vi "donut_fitting_particle(subVI).vi"(5 "Edge Options":T3={"Edge Polarity"=0, "Kernel Size"=3, "Width"=3, "Minimum Edge Strength"=10.0, "Interpolation Type"=enum."Bilinear Fixed", "Data Processing Method"=enum."Average"} {"Edge Polarity" items=["All Edges", "Rising Edges", "Falling Edges"]; "Minimum Edge Strength" format="%.2f"; "Width" step=2; "Kernel Size" step=2}, 8 "error in (no error)":errorcluster, 10 "Image Dst":T1, 11 "Image Src":T1) -> (0 "error out":errorcluster, 1 "First Edges":T2[][](array[typedef]) {"Distance (Real-World)" format="%.2f"; "Location (Real-World)"."Y" format="%.2g"; "Location (Real-World)"."X" format="%.2f"; "Noise" format="%.2f"; "Location (Pixel)"."Y" format="%.2g"; "Location (Pixel)"."X" format="%.2f"; "Strength" format="%.2f"; "Distance (Pixel)" format="%.2f"}, 2 "Last Edges":T2[][](array[typedef]) {"Distance (Real-World)" format="%.2f"; "Location (Real-World)"."Y" format="%.2g"; "Location (Real-World)"."X" format="%.2f"; "Noise" format="%.2f"; "Location (Pixel)"."Y" format="%.2g"; "Location (Pixel)"."X" format="%.2f"; "Strength" format="%.2f"; "Distance (Pixel)" format="%.2f"}, 3 "Image":T1(plugin-control))   [LabVIEW 2020]
doc: "Trova i donut all'interno dell'immagine. Fornisce in uscita informazioni sui first e last edges"
uses:
  <vilib>/vision/Image Controls.llb/IMAQ Image.ctl
  <vilib>/vision/Measure.llb/Edge Options.ctl
  <vilib>/vision/Measure.llb/Edge Polarity.ctl
  <vilib>/vision/Measure.llb/Edge New.ctl
  <vilib>/vision/NI_Vision_Development_Module.lvlib
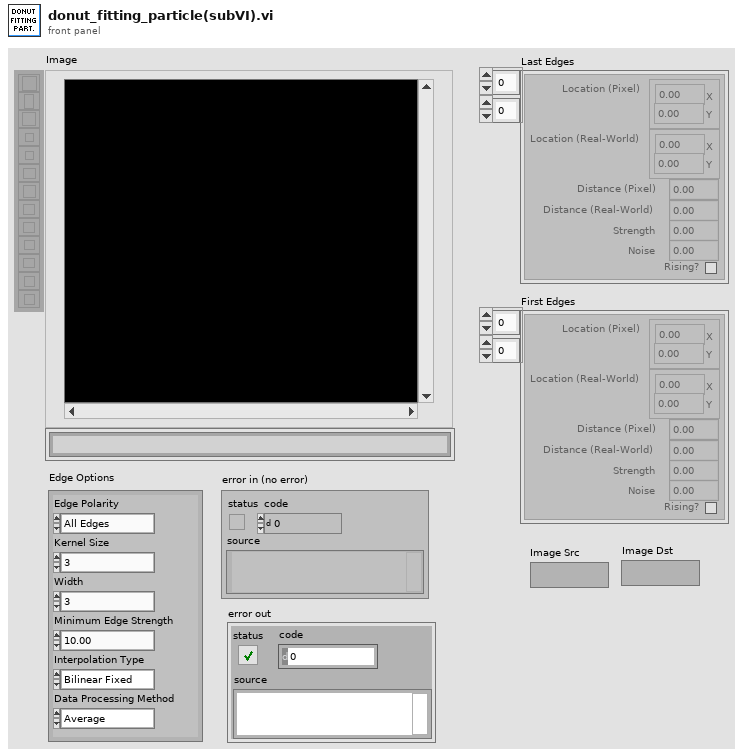
[diagram p1: front panel]
types:
  T1 = typedef "IMAQ Image.ctl" = refnum<image>
  T2 = typedef "Edge New.ctl" = cluster{"Location (Pixel)":cluster{"X":sgl, "Y":sgl}, "Location (Real-World)":cluster{"X":sgl, "Y":sgl}, "Distance (Pixel)":dbl, "Distance (Real-World)":dbl, "Strength":dbl, "Noise":dbl, "Rising?":bool}
  T3 = typedef "Edge Options.ctl" = cluster{"Edge Polarity":T4, "Kernel Size":u32, "Width":u32, "Minimum Edge Strength":sgl, "Interpolation Type":enum32{"Zero Order", "Bilinear", "Quadratic", "Cubic", "Bilinear Fixed"}, "Data Processing Method":enum32{"Average", "Median"}}
  T4 = typedef "Edge Polarity.ctl" = u32
  T5 = typedef "IMAQ Circle" = cluster{"Center X":i32, "Center Y":i32, "Inner Radius":i32, "Outer Radius":i32, "Start Angle":dbl, "End Angle":dbl}
  T6 = cluster{"Area":dbl, "Number of Holes":dbl, "Bounding Rect":cluster{"Left":dbl, "Top":dbl, "Right":dbl, "Bottom":dbl}, "Center of Mass":cluster{"X":dbl, "Y":dbl}, "Orientation":dbl, "Dimensions":cluster{"Width":dbl, "Height":dbl}}[]
  T7 = cluster{"Left":dbl, "Top":dbl, "Right":dbl, "Bottom":dbl}
  T8 = typedef "ROI Descriptor" = cluster{"Global Rectangle":i32[], "Contours":cluster{"ID":enum32{"External", "Internal"}, "Type":u32, "Coordinates":i32[]}[]}
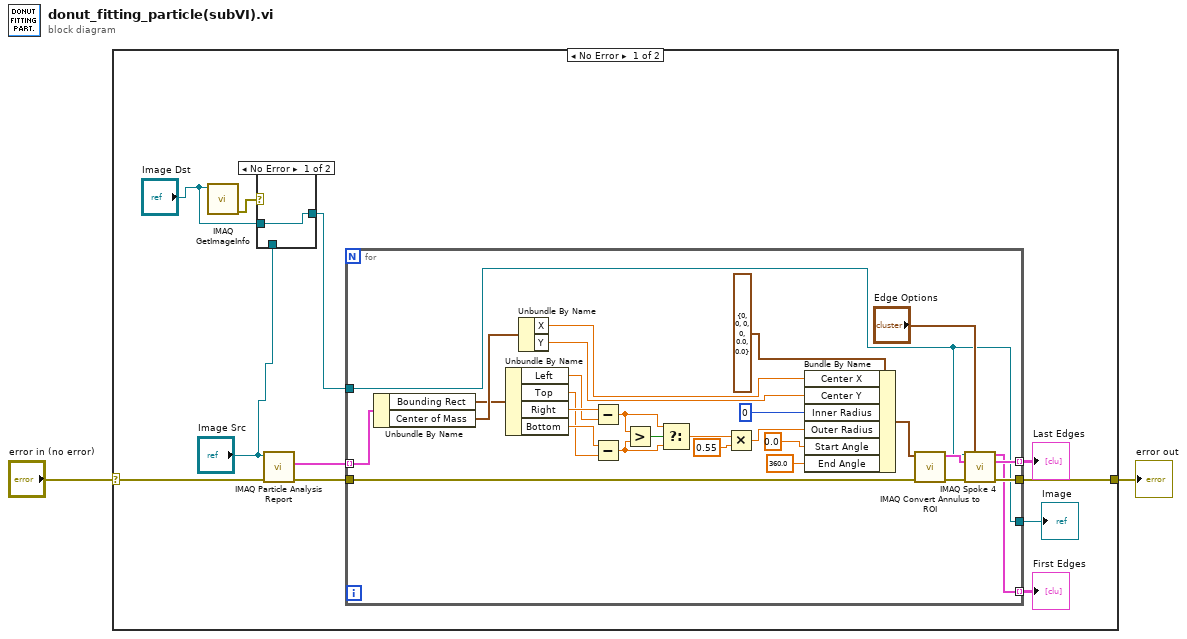
[diagram p0: block diagram]
diagram:
  n1 = case shown="No Error" "error in (no error)" {
    selector: "error in (no error)" -> [w9 w44]
    tunnel: [w11 w44] -> w2
    frame No Error {
      n2 = call "IMAQ GetImageInfo"("Image"="Image Dst") -> ("error out"=w5:errorcluster)  [unwired: 3 in, 7 out]
      n3 = case shown="No Error" w5 {
        tunnel: [w14 w15] -> w3
        tunnel: "Image Src" -> [_ w15]
        tunnel: "Image Dst" -> [w14 _]
        frame No Error {
        }
        frame Error {
        }
      }
      n4 = call "IMAQ Particle Analysis Report"("error in (no error)"=w9, "Image"="Image Src") -> ("error out"=w12:errorcluster, "Particle Reports (Pixels)"=w13:T6)  [unwired: 4 in, 4 out]
      n5 = for {
        tunnel: w13 -> [w43] mode=indexing
        tunnel: w12 -> [w16]
        tunnel: [w40] -> w11
        tunnel: [w39] -> w8 mode=indexing
        tunnel: [w38] -> w7 mode=indexing
        tunnel: w3 -> [w20]
        tunnel: [w20] -> w10
        n6 = Unbundle By Name(w43) -> ("Bounding Rect"=w21:T7, "Center of Mass"=w37:cluster{"X":dbl, "Y":dbl})
        n7 = Unbundle By Name(w21) -> ("Left"=w29:dbl, "Top"=w27:dbl, "Right"=w30:dbl, "Bottom"=w28:dbl)
        n8 = Unbundle By Name(w37) -> ("X"=w19:dbl, "Y"=w18:dbl)
        n9 = Subtract(x=w30, y=w29) -> (x-y=w25:dbl)
        n10 = Subtract(x=w28, y=w27) -> (x-y=w24:dbl)
        n11 = Greater?(x=w25, y=w24) -> (0:w26:bool)
        n12 = Select(t=w25, s=w26, f=w24) -> (s? t:f=w23:dbl)
        n13 = Multiply(x=w23, y=0.55) -> (x*y=w17:dbl)
        n14 = Bundle By Name(cluster=T5 {"Center X"=0, "Center Y"=0, "Inner Radius"=0, "Outer Radius"=0, "Start Angle"=0.0, "End Angle"=0.0} ("Annulus"), "Center X"=w19, "Center Y"=w18, "Inner Radius"=0, "Outer Radius"=w17, "Start Angle"=0.0, "End Angle"=360.0) -> (w35:T5)
        n15 = call "IMAQ Convert Annulus to ROI"("error in (no error)"=w16, "Annulus"=w35) -> ("error out"=w41:errorcluster, "ROI Descriptor"=w42:T8)  [unwired: 7 in]
        n16 = call "IMAQ Spoke 4"("Image"=w20, "Edge Options"="Edge Options", "ROI Descriptor"=w42, "error in (no error)"=w41) -> ("First Edges"=w38:T2[], "Last Edges"=w39:T2[], "error out"=w40:errorcluster)  [unwired: 8 in, 1 out]
      }
      "Image" <- w10
      "Last Edges" <- w8
      "First Edges" <- w7
    }
    frame Error {
    }
  }
  "error out" <- w2
